vi "use certificate chain data.vi"(8 "error in":errorcluster, 10 "certificate chain":string, 11 "connection creator in":refnum<class "connection creator.lvclass">) -> (0 "error out":errorcluster)   [LabVIEW 2016, in "connection creator.lvclass"]
uses:
  connection creator.lvclass
  connection creator.lvclass/connection creator.ctl
  dllwrapper/async tls dl.lvlib
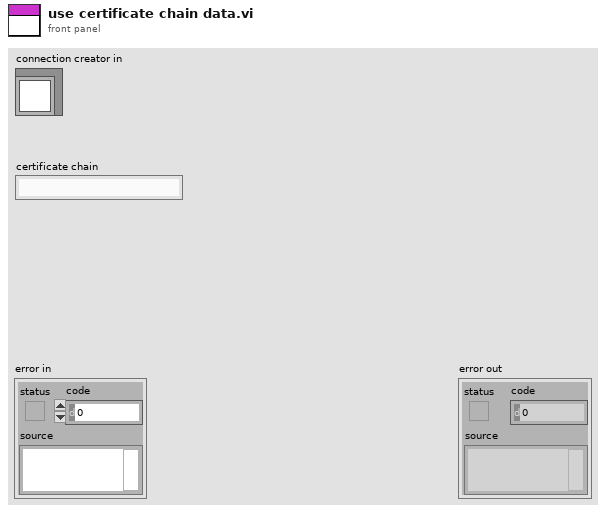
[diagram p1: front panel]
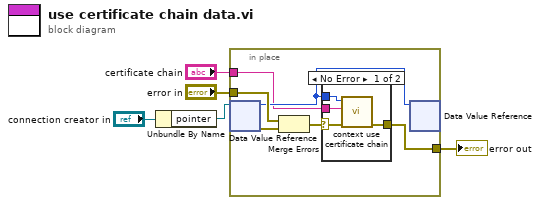
[diagram p0: block diagram]
diagram:
  n1 = Unbundle By Name("connection creator in") -> ("pointer"=w3:refnum<data-value>)
  n2 = in-place {
    in-place-border: "error in" -> [w10]
    in-place-border: [w8] -> w2
    in-place-border: "certificate chain" -> [w6]
    n3 = in-place-dvr #1(w3) -> (w7:u64, w11:errorcluster)
    n4 = Merge Errors(w10, w11) -> (w9:errorcluster)
    n5 = case shown="No Error" w9 {
      selector: w9 -> [w15 w16]
      tunnel: [w13 w16] -> w8
      tunnel: w7 -> [w14 _]
      tunnel: w6 -> [w12 _]
      frame No Error {
        n6 = call "context use certificate chain.vi"("error in"=w15, "chain"=w12, "connector"=w14) -> ("error out"=w13:errorcluster)  [unwired: 8 in]
      }
      frame Error {
      }
    }
    n7 = in-place-dvr #1(w7) -> ()  [unwired: 2 out]
  }
  "error out" <- w2
